vi "init.vi"(8 "error in (no error)":errorcluster, 9 "Duty Cycle":T1=50.0, 10 "Inputs to Periodic Wave":T2={"Frequency"=10.0, "Amplitude"=1.0, "Phase"=0.0, " Time"=0.0}, 11 "Square Wave in":refnum<class "SquareWave.lvclass">) -> (0 "error out":errorcluster, 3 "Square Wave out":refnum<class "SquareWave.lvclass">)   [LabVIEW 2015, in "SquareWave.lvclass"]
uses:
  SquareWave.lvclass
  Typedefs/PeriodicWaveInputs.ctl
  Typedefs/DutyCycle.ctl
  Typedefs/FAMTTypedefs.lvlib
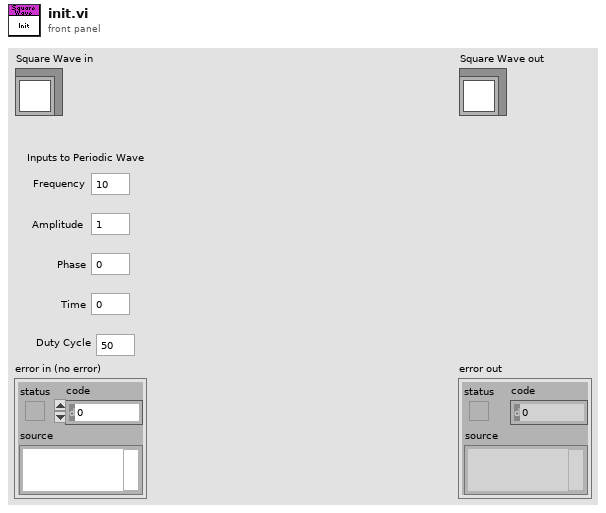
[diagram p1: front panel]
types:
  T1 = typedef "FAMTTypedefs.lvlib/DutyCycle.ctl" = dbl
  T2 = typedef "FAMTTypedefs.lvlib/PeriodicWaveInputs.ctl" = cluster{"Frequency":dbl, "Amplitude":dbl, "Phase":dbl, " Time":dbl}
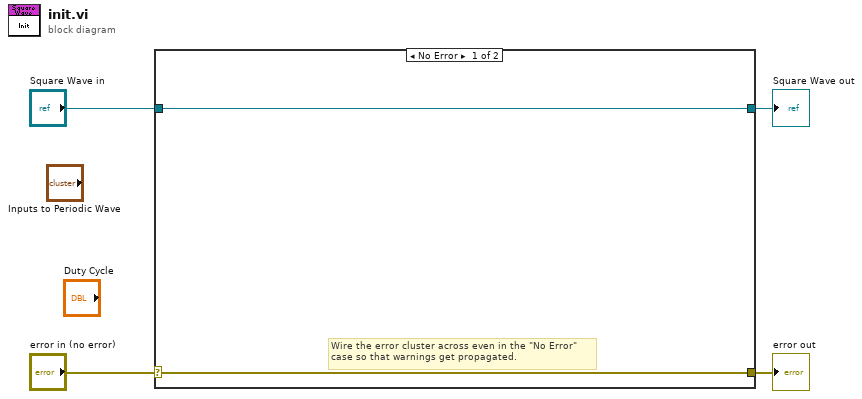
[diagram p0: block diagram]
diagram:
  n1 = case shown="No Error" "error in (no error)" {
    selector: "error in (no error)" -> [w5 w8]
    tunnel: [w5 w8] -> w3
    tunnel: [w6 w7] -> w1
    tunnel: "Square Wave in" -> [w6 w7]
    frame No Error {
      # "Wire the error cluster across even in the \"No Error\"\ncase so that warnings get propagated."
    }
    frame Error {
    }
  }
  "error out" <- w3
  "Square Wave out" <- w1
